vi "Add to Type Map.vi"(8 "error in (no error)":errorcluster, 9 ".NET AdsDataType":refnum<k24>, 10 "Type Name":string, 11 "TwinCAT ADS in":refnum<class "TwinCAT ADS.lvclass">) -> (0 "error out":errorcluster, 2 "Success?":bool, 3 "TwinCAT ADS out":refnum<class "TwinCAT ADS.lvclass">)   [LabVIEW 2018, in "TwinCAT ADS.lvclass"]
uses:
  TwinCAT ADS.lvclass
  TwinCAT.Ads
  TwinCAT ADS.lvclass/TwinCAT ADS.ctl
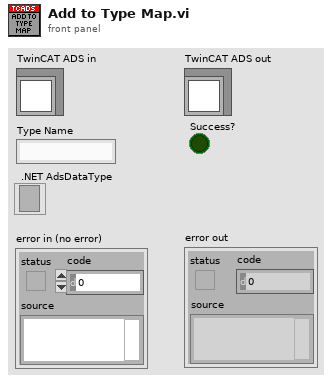
[diagram p1: front panel]
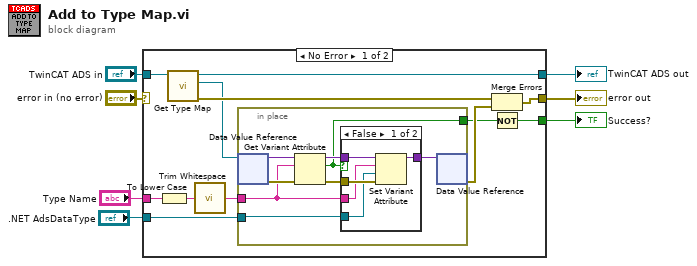
[diagram p0: block diagram]
diagram:
  n1 = case shown="No Error" "error in (no error)" {
    selector: "error in (no error)" -> [_ w34]
    tunnel: "TwinCAT ADS in" -> [w13 w35]
    tunnel: ".NET AdsDataType" -> [w19 _]
    tunnel: "Type Name" -> [w18 _]
    tunnel: [w12 w35] -> w5
    tunnel: [w16 w34] -> w4
    tunnel: [w8 _] -> w1
    frame No Error {
      n2 = To Lower Case(string=w18) -> (all lower case string=w15:string)
      n3 = call "Get Type Map.vi"("TwinCAT ADS in"=w13) -> ("error out"=w11:errorcluster, "Type Map"=w10:refnum<data-value>, "TwinCAT ADS out"=w12:refnum<class "TwinCAT ADS.lvclass">)  [unwired: 8 in]
      n4 = call <vilib>:"Trim Whitespace.vi"("string"=w15) -> ("trimmed string"=w14:string)  [unwired: 1 in]
      n5 = in-place {
        in-place-border: w19 -> [w22]
        in-place-border: w14 -> [w21]
        in-place-border: [w20] -> w9
        n6 = in-place-dvr #1(w10) -> (w26:variant, w27:errorcluster)
        n7 = Get Variant Attribute(Variant=w26, name=w21, error in=w27) -> (duplicate Variant=w25:variant, found=w20:bool, error out=w23:errorcluster)  [unwired: 1 in, 1 out]
        n8 = case shown="False" w20 {
          tunnel: w25 -> [w32 w33]
          tunnel: [w31 w33] -> w24
          tunnel: w23 -> [w30 _]
          tunnel: w22 -> [w28 _]
          tunnel: w21 -> [w29 _]
          frame False {
            n9 = Set Variant Attribute(Variant=w32, name=w29, value=w28, error in=w30) -> (Variant out=w31:variant)  [unwired: 2 out]
          }
          frame True {
          }
        }
        n10 = in-place-dvr #1(w24) -> (w17:errorcluster)  [unwired: 1 out]
      }
      n11 = Merge Errors(w11, w17) -> (w16:errorcluster)
      n12 = Not(x=w9) -> (.not. x?=w8:bool)
    }
    frame Error {
    }
  }
  "error out" <- w4
  "TwinCAT ADS out" <- w5
  "Success?" <- w1
